vi "HP 11713A.vi"(0 "VISA_IN":refnum<visa-resource-name>="GPIB0::29::INSTR", 11 "error in":errorcluster, 13 "9":bool=TRUE, 14 "0":bool=TRUE) -> (4 "visa_out":refnum<visa-resource-name>, 15 "error out":errorcluster)   [LabVIEW 2018]
doc: "HP 11713A ATTENUATOR/SWITCH DRIVER\n\nGPIB PROGRAMMING NOTES: The format of a control command consists of two ASCII characters representing the on/off status of the switch (The first character is a number designating a particular switch. The second character represents the on/off condition). There are no separators used in the command string. Data is sent with an EOI terminator (GPIB Write Mode 0). A front panel LED will activate when the instrument is put in the Remote mode. The GPIB address switch is available on the rear panel of the instrument. The 11713 is a listen only device and will not return a serial poll responce or data. Further description of the GPIB is given in section 3 of the Operating and Service manual.\n\nINTERACTIVE OPERATION: The HP 11713A Virtual Instrument (VI) provides remote control and setup of attenuators and RF coaxial switches. The VI front panel is set up in the same manner as the HP 11713A in order to add ease to programming the attenuators and configuring the coaxial switches. The panel consists of ten switches: the first four control the X attenuator, the second four control the Y attenuator, the last two provide setup for the coaxial switches. Consult the Operations Manual on page 3-11 for the attenuator programming tables. In order to operate the VI, look up the desired attenuation value in the table and set the appropriate driver switches on or off. (All of the switches are pushed in -on- as default). If coaxial switches are used, hook them up according to the manual. Once the switches are set, run the VI. The HP 11713A panel switches will verify operation (The switch LED will light in the on state. The LED is off for the off state).\n\nPROGRAMMATIC OPERATION: An example program is included in this package showing the 'HP 11713A' used programmatically. The following values can be used as inputs to the 'HP 11713A' ICON; the ICON and connector pane are shown below:\n\n \n\nGPIB ADDRESS: 28\n\nATTENUATOR X (1-4): BINARY SWITCH DEFAULT: ON\n\nATTENUATOR Y (5-8): BINARY SWITCH DEFAULT: ON\n\nSWITCHES (9,0): BINARY SWITCH DEFAULT: ON"
panel:
  in  "8":bool=TRUE
  in  "7":bool=TRUE
  in  "6":bool=TRUE
  in  "5":bool=TRUE
  in  "4":bool=TRUE
  in  "3":bool=TRUE
  in  "2":bool=TRUE
  in  "1":bool=TRUE
  # "attenuator X"
  # "switches"
  # "attenuator Y"
  # "ON\nOFF"
  # "© Copyright 1993 National Instruments Corporation.  ALL RIGHTS RESERVED."
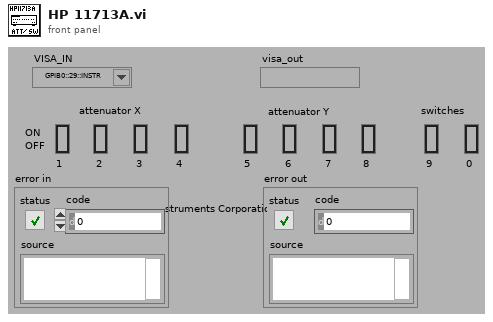
[diagram p1: front panel]
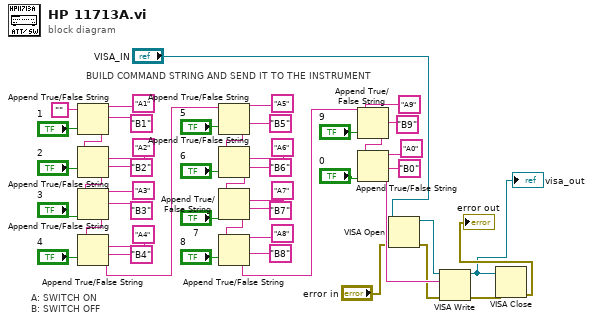
[diagram p0: block diagram]
diagram:
  # "BUILD COMMAND STRING AND SEND IT TO THE INSTRUMENT"
  # "A: SWITCH ON\nB: SWITCH OFF"
  n1 = Append True/False String(1:"1", 2:"B1", 3:"A1", 4:"") -> (0:w9:string)
  n2 = Append True/False String(1:"2", 2:"B2", 3:"A2", 4:w9) -> (0:w10:string)
  n3 = Append True/False String(1:"3", 2:"B3", 3:"A3", 4:w10) -> (0:w11:string)
  n4 = Append True/False String(1:"4", 2:"B4", 3:"A4", 4:w11) -> (0:w17:string)
  n5 = Append True/False String(1:"5", 2:"B5", 3:"A5", 4:w17) -> (0:w22:string)
  n6 = Append True/False String(1:"6", 2:"B6", 3:"A6", 4:w22) -> (0:w23:string)
  n7 = Append True/False String(1:"7", 2:"B7", 3:"A7", 4:w23) -> (0:w24:string)
  n8 = Append True/False String(1:"8", 2:"B8", 3:"A8", 4:w24) -> (0:w25:string)
  n9 = Append True/False String(1:"9", 2:"B9", 3:"A9", 4:w25) -> (0:w28:string)
  n10 = Append True/False String(1:"0", 2:"B0", 3:"A0", 4:w28) -> (0:w8:string)
  n11 = VISA Open(error in (no error)="error in", VISA resource name="VISA_IN") -> (VISA resource name=w6:refnum<visa-resource-name>, error out=w3:errorcluster)  [unwired: 3 in]
  n12 = VISA Write(VISA resource name=w6, write buffer=w8, error in (no error)=w3) -> (VISA resource name out=w1:refnum<visa-resource-name>, error out=w7:errorcluster)  [unwired: 1 out]
  "visa_out" <- w1
  n13 = VISA Close(VISA resource name=w1, error in (no error)=w7) -> (error out=→"error out":errorcluster)
